vi "Build FEFF Filter Query.vi"(5 "ORDER BY needed?(Yes)":bool=TRUE, 7 "WHERE needed?(Yes)":bool=TRUE, 8 "Stop Test Cycle":string(combo), 9 "Start Test Cycle":string(combo), 10 "Test Mode":string(combo), 11 "Test Socket":string(combo)) -> (3 "String":string)   [LabVIEW 2023, in "Data Analysis.lvlib"]
uses:
  Data Analysis.lvlib
  <vilib>/Utility/error.llb/Trim Whitespace One-Sided.vi
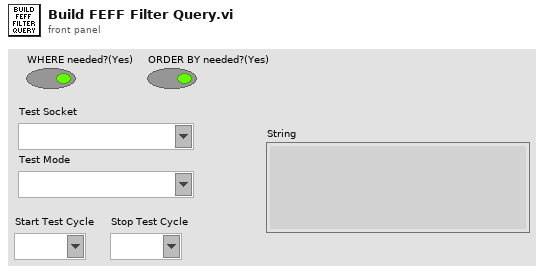
[diagram p1: front panel]
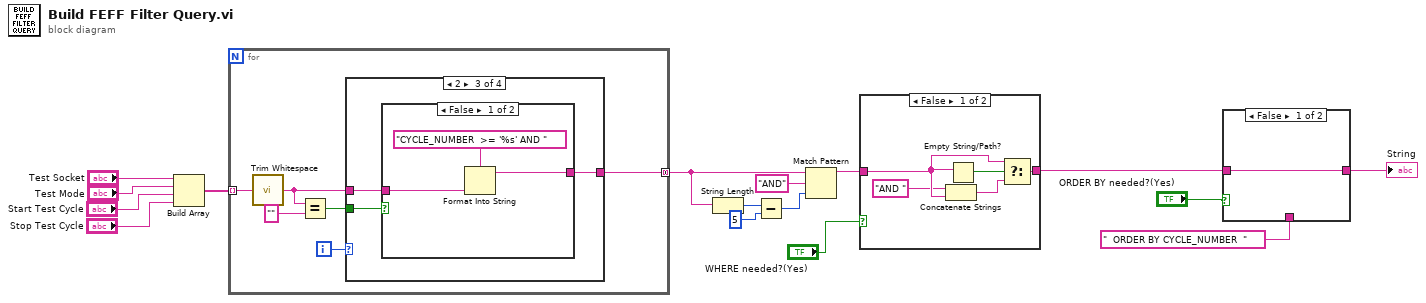
[diagram p0: block diagram]
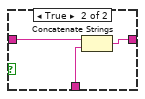
[diagram p2: hidden frame]
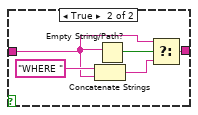
[diagram p3: hidden frame]
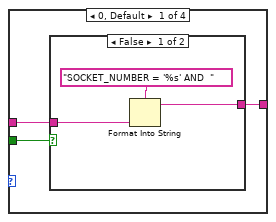
[diagram p4: hidden frame]
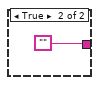
[diagram p5: hidden frame]
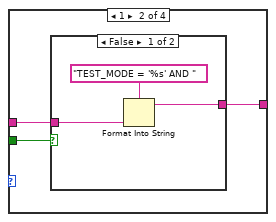
[diagram p6: hidden frame]
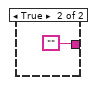
[diagram p7: hidden frame]
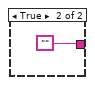
[diagram p8: hidden frame]
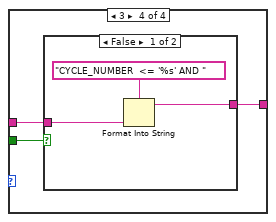
[diagram p9: hidden frame]
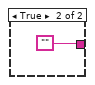
[diagram p10: hidden frame]
diagram:
  n1 = Build Array("Test Socket", "Test Mode", "Start Test Cycle", "Stop Test Cycle") -> (w14:string[])
  n2 = for {
    tunnel: w14 -> [w22] mode=indexing
    tunnel: [w17] -> w8 mode=concatenating
    i -> [w20]
    n3 = call <vilib>:"Trim Whitespace.vi"("string"=w22) -> ("trimmed string"=w19:string)  [unwired: 1 in]
    n4 = Equal?(x=w19, y="") -> (x = y?=w18:bool)
    n5 = case shown="2" w20 {
      tunnel: w19 -> [w24 w31 w38 w45]
      tunnel: w18 -> [w25 w32 w39 w46]
      tunnel: [w23 w30 w37 w44] -> w17
      frame 0, Default {
        n6 = case shown="False" w25 {
          tunnel: w24 -> [w27 _]
          tunnel: [w26 ""] -> w23
          frame False {
            n7 = Format Into String(format string="SOCKET_NUMBER = '%s' AND  ", w27) -> (resulting string=w26:string)  [unwired: 2 in, 1 out]
          }
          frame True {
          }
        }
      }
      frame 1 {
        n8 = case shown="False" w32 {
          tunnel: w31 -> [w34 _]
          tunnel: [w33 ""] -> w30
          frame False {
            n9 = Format Into String(format string="TEST_MODE = '%s' AND ", w34) -> (resulting string=w33:string)  [unwired: 2 in, 1 out]
          }
          frame True {
          }
        }
      }
      frame 2 {
        n10 = case shown="False" w39 {
          tunnel: w38 -> [w41 _]
          tunnel: [w40 ""] -> w37
          frame False {
            n11 = Format Into String(format string="CYCLE_NUMBER  >= '%s' AND ", w41) -> (resulting string=w40:string)  [unwired: 2 in, 1 out]
          }
          frame True {
          }
        }
      }
      frame 3 {
        n12 = case shown="False" w46 {
          tunnel: w45 -> [w48 _]
          tunnel: [w47 ""] -> w44
          frame False {
            n13 = Format Into String(format string="CYCLE_NUMBER  <= '%s' AND ", w48) -> (resulting string=w47:string)  [unwired: 2 in, 1 out]
          }
          frame True {
          }
        }
      }
    }
  }
  n14 = String Length(string=w8) -> (length=w7:i32)
  n15 = Subtract(x=w7, y=5) -> (x-y=w5:i32)
  n16 = Match Pattern(string=w8, regular expression="AND", offset (0)=w5) -> (before substring=w9:string)  [unwired: 3 out]
  n17 = case shown="False" "WHERE needed?(Yes)" {
    tunnel: [w53 w57] -> w13
    tunnel: w9 -> [w52 w56]
    frame False {
      n18 = Concatenate Strings("AND ", w52) -> (w54:string)
      n19 = Empty String/Path?(string/path=w52) -> (empty?=w55:bool)
      n20 = Select(t=w52, s=w55, f=w54) -> (s? t:f=w53:string)
    }
    frame True {
      n21 = Concatenate Strings("WHERE ", w56) -> (w58:string)
      n22 = Empty String/Path?(string/path=w56) -> (empty?=w60:bool)
      n23 = Select(t=w56, s=w60, f=w58) -> (s? t:f=w57:string)
    }
  }
  n24 = case shown="False" "ORDER BY needed?(Yes)" {
    tunnel: w13 -> [w61 w64]
    tunnel: "  ORDER BY CYCLE_NUMBER  " -> [_ w63]
    tunnel: [w61 w62] -> w11
    frame False {
    }
    frame True {
      n25 = Concatenate Strings(w64, w63) -> (w62:string)
    }
  }
  "String" <- w11
